vi "Goal-directed Line Following.vi"() -> ()   [LabVIEW 2019]
uses:
  SubVIs/GDLF SM States.ctl
  <vilib>/Platform/TimedLoop/XDataNode/timing_clust.ctl
  <vilib>/Platform/TimedLoop/XDataNode/nitl_modes.ctl
  <vilib>/Platform/TimedLoop/XDataNode/wakeup.ctl
  <extravilib>/ChannelInstances/Tag-bool/Write With Abort.vi
  <extravilib>/ChannelInstances/Tag-a[.](dbl)/Read With Abort.vi
  <extravilib>/ChannelInstances/Tag-a[.](dbl)/Write With Abort.vi
  <extravilib>/ChannelInstances/Tag-bool/Read With Abort.vi
  <extravilib>/ChannelInstances/Tag-dbl/Write With Abort.vi
  <extravilib>/ChannelInstances/Lossy Stream-a[.,.](dbl)/Read With Abort.vi
  <extravilib>/ChannelInstances/Tag-dbl/Read With Abort.vi
  <extravilib>/ChannelInstances/Lossy Stream-a[.,.](dbl)/Write With Abort.vi
  <extravilib>/ChannelInstances/Lossy Stream-a[.,.](dbl)/EndpointRead.vi
  <extravilib>/ChannelInstances/Lossy Stream-a[.,.](dbl)/Endpoint.vi
  <extravilib>/ChannelInstances/Tag-bool/Instantiate.vi
  <extravilib>/ChannelInstances/Tag-dbl/Instantiate.vi
  <extravilib>/ChannelInstances/Lossy Stream-a[.,.](dbl)/Instantiate.vi
  <extravilib>/ChannelInstances/Tag-a[.](dbl)/Instantiate.vi
  <extravilib>/ChannelInstances/Tag-bool/EndpointRead.vi
  <extravilib>/ChannelInstances/Tag-a[.](dbl)/EndpointRead.vi
  <extravilib>/ChannelInstances/Tag-dbl/EndpointRead.vi
  <extravilib>/ChannelInstances/Lossy Stream-a[.,.](dbl)/)Channel.vi
  <extravilib>/ChannelInstances/Tag-bool/Endpoint.vi
  <extravilib>/ChannelInstances/Tag-a[.](dbl)/Endpoint.vi
  <extravilib>/ChannelInstances/Tag-dbl/Endpoint.vi
  <resource>/ChannelSupport/_ChannelSupport/WaitIfNeeded.vi
  <vilib>/Platform/TimedLoop/XDataNode/XDataNode.xnode
  <extravilib>/ChannelInstances/Tag-bool.lvlib
  <vilib>/Platform/TimedLoop/XDataNode/XDNodeRunTimeDep.lvlib
  <extravilib>/ChannelInstances/Tag-a[.](dbl).lvlib
  <extravilib>/ChannelInstances/Lossy Stream-a[.,.](dbl).lvlib
  <extravilib>/ChannelInstances/Tag-dbl.lvlib
panel:
  in  "Hue Threshold":cluster{i32, i32}(slide)={0, 255} scale=0.0..255.0
  in  "Saturation Threshold":cluster{i32, i32}(slide)={0, 255} scale=0.0..255.0
  in  "Luminance Threshold":cluster{i32, i32}(slide)={0, 255} scale=0.0..255.0
  out "error out":errorcluster
  out "System State":T1
  out "Destination Task \nCoordinates (cm)":dbl[](array[numeric])
  in  "Stop Button":bool
  out "Calibrated":bool
  out "Information":string
  in  "GO?":bool
  out "Processed Image":T2(plugin-control)
  out "Desired Task \nCoordinates (cm)":dbl[](array[numeric])
  out "Current Task Coordinates (cm)":dbl[](array[numeric])
  out "Silk":T2(plugin-control)
  out "Original Acquired Image":T2(plugin-control)
  # "Mechatronic Systems Board"
  # "Goal-directed Line Following"
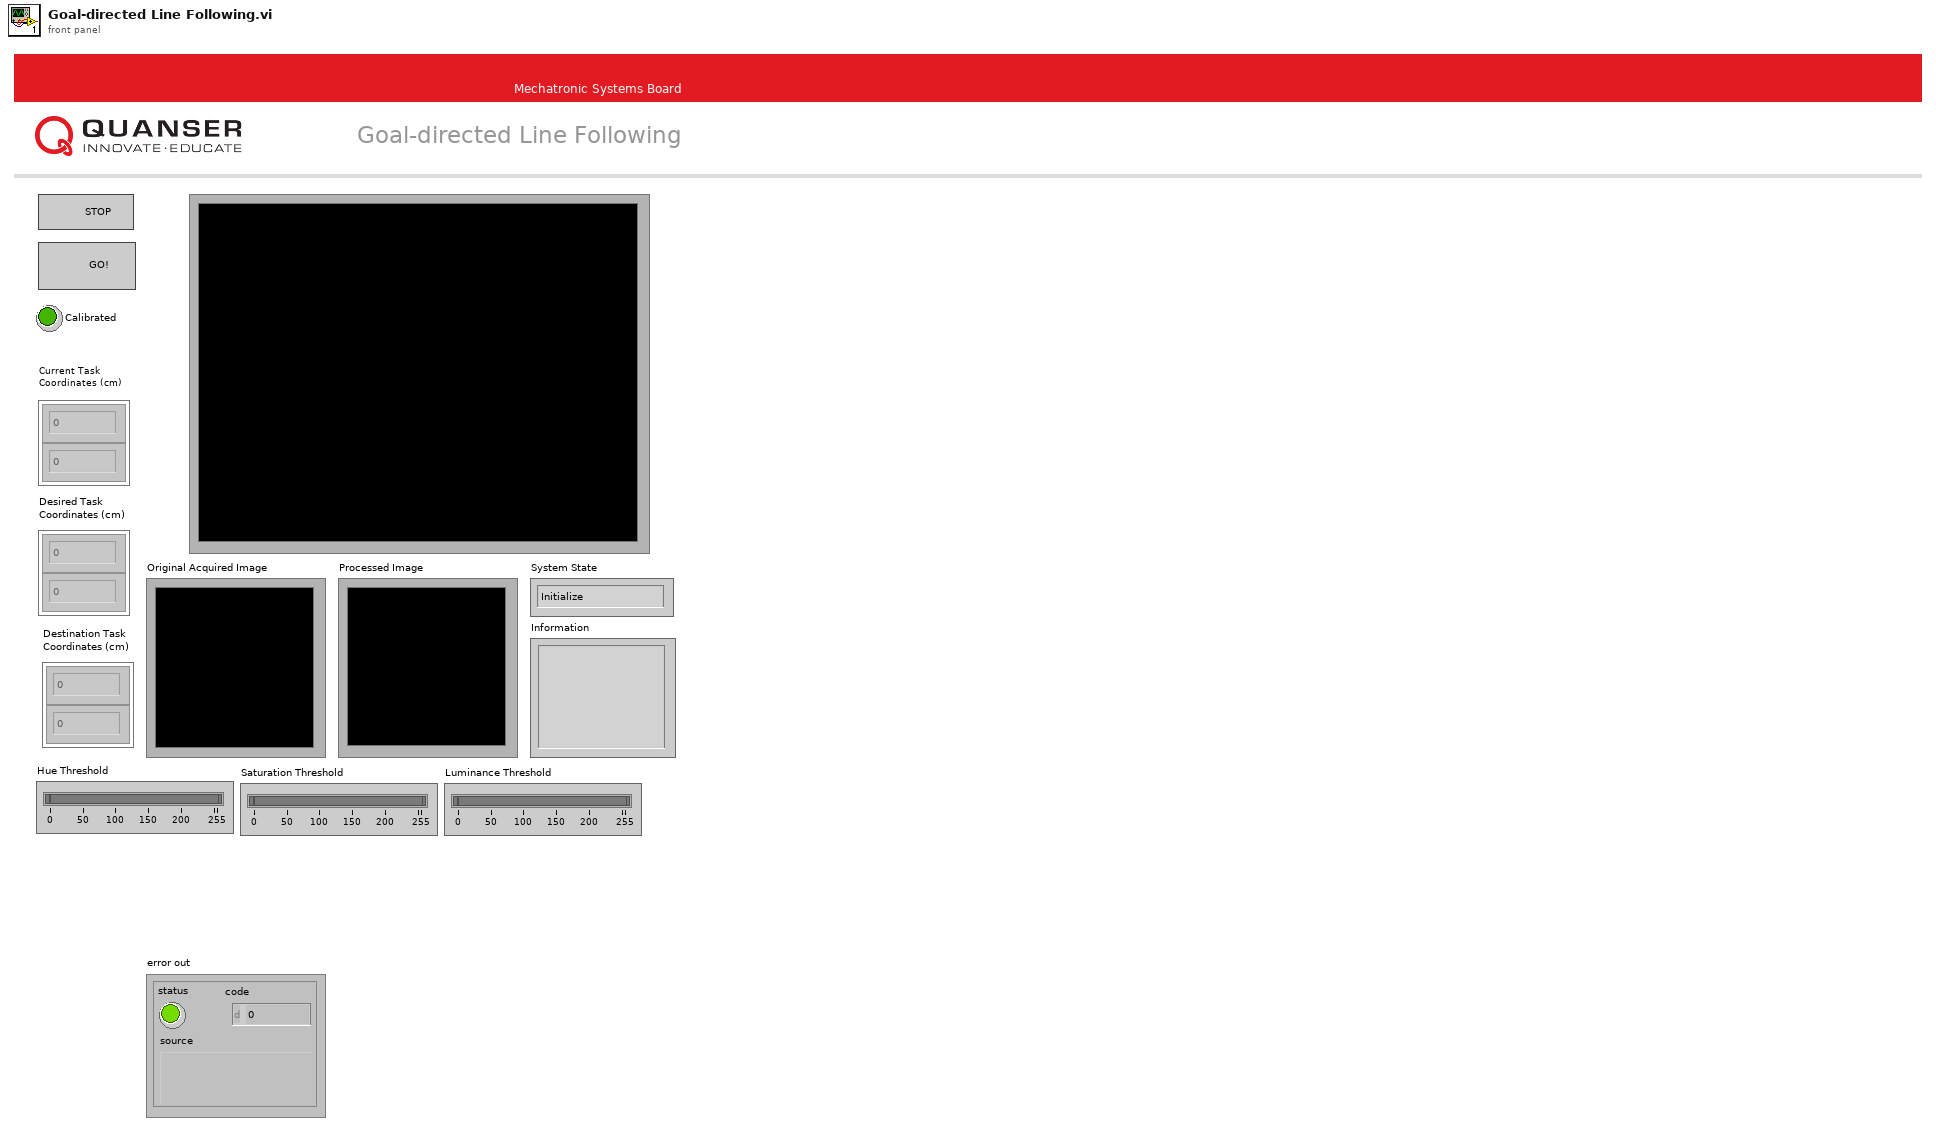
[diagram p1: front panel]
types:
  T1 = typedef "GDLF SM States.ctl" = enum16{"Initialize", "Set Destination", "Move", "Wait", "Backtrack", "Stop"}
  T2 = typedef "IMAQ Image.ctl" = refnum<image>
  T3 = typedef "QNET MS IO Cluster.ctl" = cluster{"Error":errorcluster, "Encoder Calibration Values":i32[], "Update Calibration":bool, "JPEG Resolutions":u16, "Raw Resolutions":u16, "Image Mode":enum16{"RAW RGB", "RAW Gray Scale", "JPEG"}, "FPGA Ref":refnum<k20>}
  T4 = typedef "XDNodeRunTimeDep.lvlib/timing_clust.ctl" = cluster{"Expected End [f-1]":u64, "Actual End [f-1]":u64, "Finished Late? [f-1]":bool, "Expected End [i-1]":u64, "Actual End [i-1]":u64, "Finished Late? [i-1]":bool, "Expected Start [i]":u64, "Actual Start [i]":u64, "Expected Start [f]":u64, "Actual Start [f]":u64, "Source Name":string, "Structure Name":string, "Period":i64, "Deadline":i64, "Offset":i64, "Start":i64, "Priority":i32, "Timeout":i32, "Mode":T5, "Wakeup Reason":T6, "Error":errorcluster, "Source Type":string, "Secondary Source Type":string, "Global End Time":u64, "Global Start Time":u64, "Frame Duration":u64, "Iteration Duration":u64, "Assigned CPU":i32, "I/O Scan Engine Mode":u32}
  T5 = typedef "XDNodeRunTimeDep.lvlib/nitl_modes.ctl" = enum32{"No Change", "Process missed periods, maintain original phase", "Discard missed periods, maintain original phase", "Process missed periods, ignore original phase", "Discard missed periods, ignore original phase"}
  T6 = typedef "XDNodeRunTimeDep.lvlib/wakeup.ctl" = enum32{"Normal", "Aborted", "Asynchronous wakeup", "Timing source error", "Timed loop error", "Timeout"}
  T7 = typedef "ROI Descriptor" = cluster{"Global Rectangle":i32[], "Contours":cluster{"ID":enum32{"External", "Internal"}, "Type":u32, "Coordinates":i32[]}[]}
  T8 = cluster{"Hue Threshold":cluster{i32, i32}, "Saturation Threshold":cluster{i32, i32}, "Luminance Threshold":cluster{i32, i32}}
  T9 = typedef "Lossy Stream-a[.,.](dbl).lvlib/)Channel.ctl" = refnum<queue>
  T10 = typedef "Tag-a[.](dbl).lvlib/))Channel.ctl" = refnum<queue>
  T11 = typedef "Tag-bool.lvlib/))Channel.ctl" = refnum<queue>
  T12 = cluster{"Global Rectangle":i32[], "Contours":cluster{"Contour Type":u32, "ROI Type":u32, "Points":i32[]}[]}
  T13 = typedef "Tag-dbl.lvlib/))Channel.ctl" = refnum<queue>
  T14 = cluster{"Contour Type":u32, "ROI Type":u32, "Points":i32[]}[]
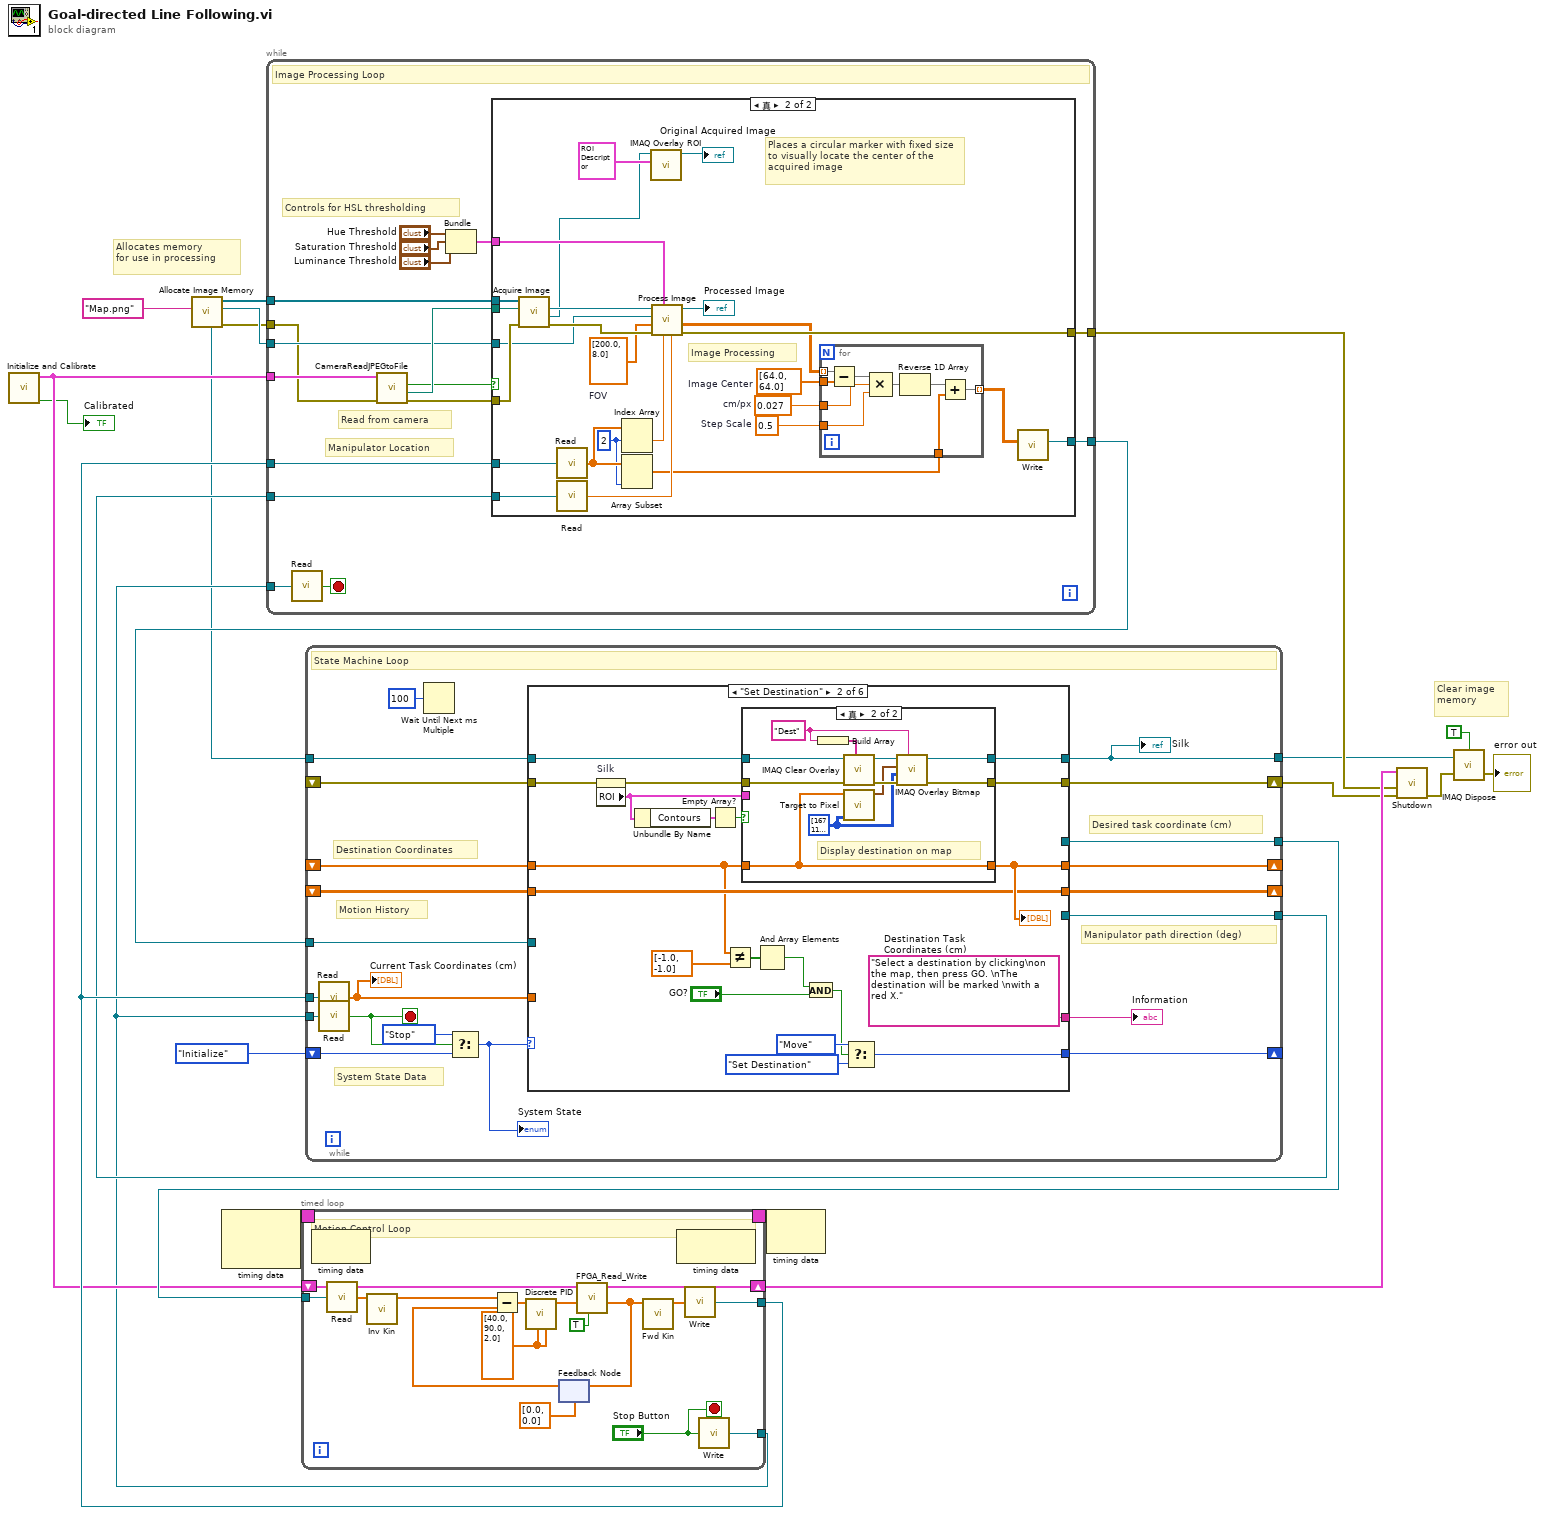
[diagram p0: block diagram]
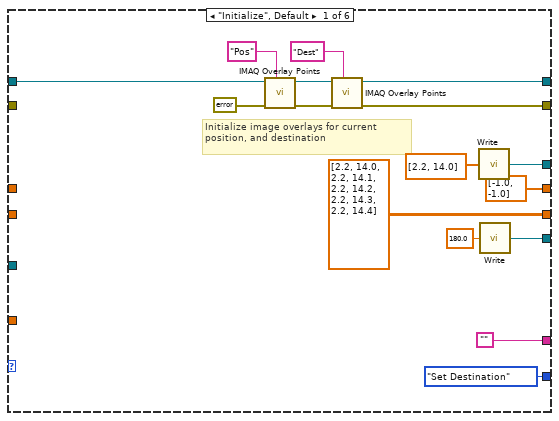
[diagram p2: hidden frame]
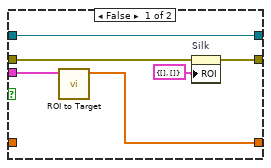
[diagram p3: hidden frame]
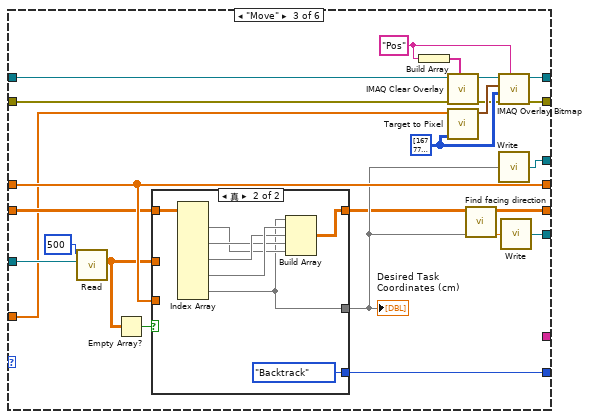
[diagram p4: hidden frame]
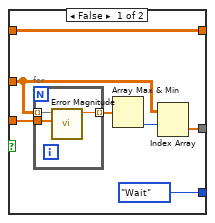
[diagram p5: hidden frame]
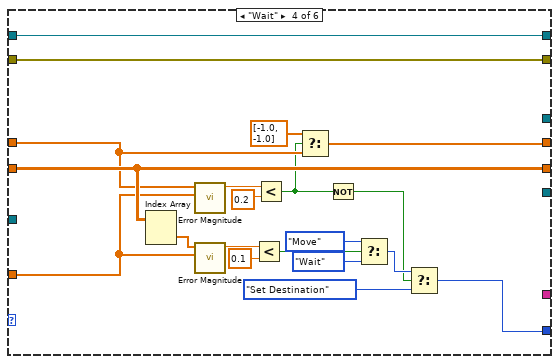
[diagram p6: hidden frame]
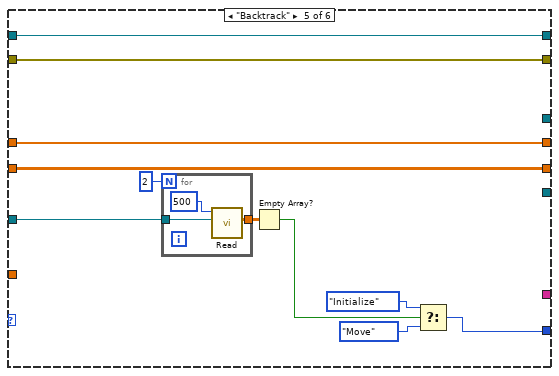
[diagram p7: hidden frame]
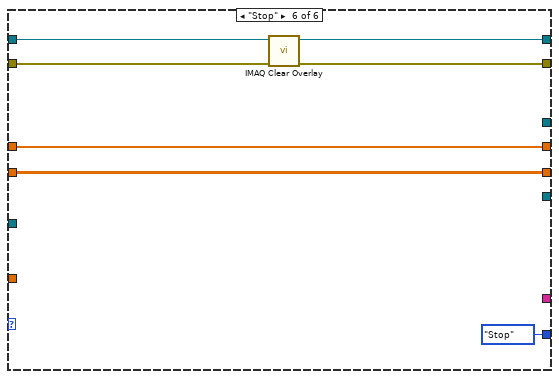
[diagram p8: hidden frame]
diagram:
  # "Allocates memory\nfor use in processing"
  # "Clear image\nmemory"
  n1 = call "Initialize and Calibrate.vi"() -> ("Calibrated"=→"Calibrated":bool, "IO Cluster"=w11:T3)  [unwired: 10 in]
  n2 = call "Allocate Image Memory.vi"("Base Image File"="Map.png") -> ("error out"=w19:errorcluster, "HSL Threshold"=w20:T2, "Acquisition Memory"=w21:T2[], "Base Image"=w2:T2)  [unwired: 5 in, 2 out]
  n3 = node-c288() -> (w18:T4)  [unwired: 2 in]
  n4 = while {
    tunnel: w11 -> [w39]
    tunnel: [w35] -> w8
    tunnel: w21 -> [w34]
    tunnel: w20 -> [w33]
    tunnel: w19 -> [w32]
    tunnel: [w31] -> w14
    tunnel: w15 -> [w29]
    tunnel: w13 -> [w30]
    tunnel: w4 -> [w28]
    stop <- w27 stop-if-true
    # "Controls for HSL thresholding"
    # "Read from camera"
    # "Manipulator Location"
    # "Image Processing Loop"
    n5 = call <extravilib>:"Read.vi"("channel"=w28) -> ("element"=w27:bool)  [unwired: 1 in, 1 out]
    n6 = call "CameraReadJPEGtoFile.vi"("error in"=w32, "IO Cluster In"=w39) -> ("Error Out"=w36:errorcluster, "Image File"=w38:path, "New Image Data"=w37:bool)  [unwired: 6 in, 1 out]
    n7 = Bundle("Hue Threshold"="Hue Threshold", "Saturation Threshold"="Saturation Threshold", "Luminance Threshold"="Luminance Threshold") -> (w23:T8)  [unwired: 1 in]
    n8 = case shown="真" w37 {
      tunnel: w38 -> [_ w64]
      tunnel: w36 -> [w40 w65]
      tunnel: [w40 w60] -> w35
      tunnel: w34 -> [_ w63]
      tunnel: w33 -> [_ w55]
      tunnel: [_ w52] -> w31
      tunnel: w30 -> [_ w46]
      tunnel: w29 -> [_ w45]
      tunnel: w23 -> [_ w44]
      frame False {
      }
      frame True {
        w50 = 2 ("index")
        w53 = 0.5  # Step Scale
        w58 = 0.027  # cm/px
        w57 = dbl[] [64.0, 64.0]  # Image Center
        w59 = dbl[] [200.0, 8.0]  # FOV
        # "Image Processing"
        # "Places a circular marker with fixed size to visually locate the center of the acquired image"
        n9 = call "Acquire Image.vi"("Error In"=w65, "File Path"=w64, "Acquisition Memory"=w63) -> ("Error Out"=w61:errorcluster, "Source Image"=w41:T2, "HSL Image"=w42:T2)  [unwired: 4 in, 2 out]
        n10 = call <extravilib>:"Read.vi"("channel"=w45) -> ("element"=w51:dbl[])  [unwired: 1 in, 1 out]
        n11 = call <extravilib>:"Read.vi"("channel"=w46) -> ("element"=w49:dbl)  [unwired: 1 in, 1 out]
        n12 = Index Array(array=w51, index #1=w50) -> (element #1=w48:dbl)  [unwired: 1 in, 1 out]
        n13 = Array Subset(array=w51, length=w50) -> (w47:dbl[])  [unwired: 1 in]
        n14 = call "IMAQ Overlay ROI"("ROI Descriptor"=T7 {"Global Rectangle"=[16, 0, 145, 129], "Contours"=[{"ID"=enum."External", "Type"=7, "Coordinates"=[64, 64, 7, 8, 0, 0]}]}, "Image"=w41) -> ("Image Out"=→"Original Acquired Image":T2)  [unwired: 8 in, 1 out]
        n15 = call "Process Image.vi"("Path Angle"=w49, "Camera Angle"=w48, 7:w44, "Error In"=w61, "FOV"=w59, "Process Memory"=w55, "Acquired Image"=w42) -> ("Error Out"=w60:errorcluster, "Particle Locations"=w56:dbl[][], "Processed Image"=→"Processed Image":T2)  [unwired: 2 in]
        n16 = for {
          tunnel: w57 -> [w75]
          tunnel: [w73] -> w54 mode=indexing
          tunnel: w56 -> [w72] mode=indexing
          tunnel: w58 -> [w71]
          tunnel: w47 -> [w68]
          tunnel: w53 -> [w67]
          n17 = Subtract(x=w72, y=w75) -> (x-y=w74:dbl[])
          n18 = Compound Arithmetic op=MULTIPLY(w74, w71, w67) -> (w70:dbl[])
          n19 = Reverse 1D Array(array=w70) -> (reversed array=w69:dbl[])
          n20 = Add(x=w69, y=w68) -> (x+y=w73:dbl[])
        }
        n21 = call <extravilib>:"Write.vi"("element"=w54) -> ("channel"=w52:T9)  [unwired: 8 in, 2 out]
      }
    }
  }
  n22 = timed-loop {
    timing: w18 -> [_]
    timing-out: [_] -> w17
    tunnel: [w82] -> w15
    tunnel: w16 -> [w81]
    shift-right: [w87] -> w12
    shift-left: w11 -> [w79]
    tunnel: [w77] -> w4
    stop <- "Stop Button" stop-if-true
    w76 = dbl[] [40.0, 90.0, 2.0] ("Gains Motor 0")
    # "Motion Control Loop"
    n23 = node-c288() -> ()  [unwired: 1 in, 1 out]
    n24 = call <extravilib>:"Read.vi"("channel"=w81) -> ("element"=w80:dbl[])  [unwired: 1 in, 1 out]
    n25 = call "Inv Kin.vi"("Task Coordinates (cm)"=w80) -> ("Joint Coordinates (rad)"=w88:dbl[])  [unwired: 10 in]
    n26 = feedback #1(dbl[] [0.0, 0.0] ("Joint Coordinates (rad)")) -> (w86:dbl[])
    n27 = Subtract(x=w88, y=w86) -> (x-y=w89:dbl[])
    n28 = call "Discrete PID.vi"("Gains Motor 1"=w76, "Gains Motor 0"=w76, "Error Array"=w89) -> ("Voltage"=w90:dbl[])  [unwired: 8 in]
    n29 = call "FPGA_Read_Write.vi"("Motors enabled?"=TRUE, "Commands"=w90, "IO Cluster In"=w79) -> ("Joint Coordinates (rad)"=w85:dbl[], "IO Cluster Out"=w87:T3)  [unwired: 5 in, 2 out]
    n30 = feedback-in #1(w85) -> ()
    n31 = call "Fwd Kin.vi"("Joint Coordinates (rad)"=w85) -> ("Task Coordinates (cm)"=w83:dbl[])  [unwired: 9 in, 1 out]
    n32 = node-c288() -> ()  [unwired: 1 in, 1 out]
    n33 = call <extravilib>:"Write.vi"("element"=w83) -> ("channel"=w82:T10)  [unwired: 1 out]
    n34 = call <extravilib>:"Write.vi"("element"="Stop Button") -> ("channel"=w77:T11)  [unwired: 1 out]
  }
  n35 = while {
    tunnel: w4 -> [w114]
    shift-right: [w112] -> _
    shift-left: _ -> [w113]
    tunnel: w14 -> [w109]
    tunnel: [w105] -> w16
    tunnel: w15 -> [w111]
    tunnel: [w106] -> w13
    tunnel: w2 -> [w104]
    shift-right: [w108] -> _
    shift-left: _ -> [w107]
    shift-right: [w103] -> _
    shift-left: GDLF_SM_States."Initialize" ("System State") -> [w101]
    shift-right: [w97] -> w9
    shift-left: _ -> [w96]
    tunnel: [w94] -> w6
    stop <- w98 stop-if-true
    # "Manipulator path direction (deg)"
    # "Destination Coordinates"
    # "Motion History"
    # "Desired task coordinate (cm)"
    # "System State Data"
    # "State Machine Loop"
    n36 = call <extravilib>:"Read.vi"("channel"=w111) -> ("element"=w110:dbl[])  [unwired: 1 in, 1 out]
    "Current Task Coordinates (cm)" <- w110
    n37 = call <extravilib>:"Read.vi"("channel"=w114) -> ("element"=w98:bool)  [unwired: 1 in, 1 out]
    n38 = Wait Until Next ms Multiple(millisecond multiple=u32 100) -> ()  [unwired: 1 out]
    n39 = Select(t=GDLF_SM_States."Stop", s=w98, f=w101) -> (s? t:f=w100:T1)
    "System State" <- w100
    n40 = case shown="\"Set Destination\"" w100 {
      tunnel: w113 -> [_ w145 w173 w226 w237 w249]
      tunnel: [dbl[][] [[2.2, 14.0], [2.2, 14.1], [2.2, 14.2], [2.2, 14.3], [2.2, 14.4]] w145 w177 w226 w237 w249] -> w112
      tunnel: w110 -> [_ _ w168 w215 _ _]
      tunnel: w107 -> [_ w137 w184 w218 w239 w248]
      tunnel: w109 -> [_ _ w191 _ w235 _]
      tunnel: [dbl[] [-1.0, -1.0] ("Joint Coordinates (rad)") w150 w184 w217 w239 w248] -> w108
      tunnel: [w127 _ w190 _ _ _] -> w106
      tunnel: [w124 _ w189 _ _ _] -> w105
      tunnel: w104 -> [w122 w144 w188 w219 w238 w247]
      tunnel: [GDLF_SM_States."Set Destination" ("System State") w149 w171 w210 w230 GDLF_SM_States."Stop" ("System State")] -> w103
      tunnel: ["" "Select a destination by clicking\non the map, then press GO. \nThe destination will be marked \nwith a red X." _ _ _ _] -> w102
      tunnel: [w117 w142 w185 w220 w240 w244] -> w97
      tunnel: w96 -> [_ w146 w187 w220 w240 w246]
      tunnel: [w119 w141 w186 w219 w238 w245] -> w94
      frame "Initialize", Default {
        # "Initialize image overlays for current\nposition, and destination"
        n41 = call "IMAQ Overlay Points"("Group"="Pos", "error in (no error)"=errorcluster {"status"=FALSE, "code"=0, "source"=""} ("error out"), "Image"=w122) -> ("error out"=w118:errorcluster, "Image Out"=w120:T2)  [unwired: 7 in]
        n42 = call "IMAQ Overlay Points"("Group"="Dest", "error in (no error)"=w118, "Image"=w120) -> ("error out"=w117:errorcluster, "Image Out"=w119:T2)  [unwired: 7 in]
        n43 = call <extravilib>:"Write.vi"("element"=dbl[] [2.2, 14.0] ("Joint Coordinates (rad)")) -> ("channel"=w124:T10)  [unwired: 1 out]
        n44 = call <extravilib>:"Write.vi"("element"=180.0) -> ("channel"=w127:T13)  [unwired: 1 out]
      }
      frame "Set Destination" {
        n45 = property on="Silk" class="ImageControl"(error in=w146) -> (error out=w143:errorcluster, "ROI"=w138:T12)  [unwired: 1 in, 1 out]
        n46 = Unbundle By Name(w138) -> ("Contours"=w139:T14)
        n47 = Empty Array?(array=w139) -> (empty?=w140:bool)
        n48 = Not Equal?(x=w137, y=dbl[] [-1.0, -1.0] ("Joint Coordinates (rad)")) -> (x != y?=w133:bool[])
        n49 = case shown="真" w140 {
          tunnel: [w151 w163] -> w150
          tunnel: w144 -> [w153 w165]
          tunnel: w143 -> [w152 w160]
          tunnel: [w155 w159] -> w142
          tunnel: [w153 w164] -> w141
          tunnel: w137 -> [_ w163]
          tunnel: w138 -> [w156 _]
          frame False {
            n50 = call "ROI to Target.vi"("ROI"=w156) -> ("Target Coordinates"=w151:dbl[])  [unwired: 8 in, 2 out]
            n51 = property on="Silk" class="ImageControl"(error in=w152, "ROI"=T12 {"Global Rectangle"=[], "Contours"=[]}) -> (error out=w155:errorcluster)  [unwired: 1 in, 1 out]
          }
          frame True {
            w158 = "Dest" ("Group")
            w161 = u32[][] [[16711680, 16711680, 16777216, 16777216, 16777216, 16777216, 16777216, 16711680, 16711680], [16711680, 16711680, 16711680, 16777216, 16777216, 16777216, 16711680, 16711680, 16711680], [16777216, 16711680, 16711680, 16711680, 16777216, 16711680, 16711680, 16711680, 16777216], [16777216, 16777216, 16711680, 16711680, 16711680, 16711680, 16711680, 16777216, 16777216], [16777216, 16777216, 16777216, 16711680, 16711680, 16711680, 16777216, 16777216, 16777216], [16777216, 16777216, 16711680, 16711680, 16711680, 16711680, 16711680, 16777216, 16777216], [16777216, 16711680, 16711680, 16711680, 16777216, 16711680, 16711680, 16711680, 16777216], [16711680, 16711680, 16711680, 16777216, 16777216, 16777216, 16711680, 16711680, 16711680], [16711680, 16711680, 16777216, 16777216, 16777216, 16777216, 16777216, 16711680, 16711680]] ("Bitmap")
            # "Display destination on map"
            n52 = Build Array(w158) -> (w157:string[])
            n53 = call "IMAQ Clear Overlay"("Groups"=w157, "error in (no error)"=w160, "Image"=w165) -> ("error out"=w166:errorcluster, "Image Out"=w167:T2)  [unwired: 7 in]
            n54 = call "Target to Pixel.vi"("Symbol"=w161, "Target Coordinates"=w163) -> ("Target Pixel"=w162:cluster{"X":i32, "Y":i32})  [unwired: 9 in]
            n55 = call "IMAQ Overlay Bitmap"("Group"=w158, "error in (no error)"=w166, "Bitmap"=w161, "Top Left Point"=w162, "Image"=w167) -> ("error out"=w159:errorcluster, "Image Out"=w164:T2)  [unwired: 5 in]
          }
        }
        "Destination Task \nCoordinates (cm)" <- w150
        n56 = And Array Elements(Boolean array=w133) -> (logical AND=w132:bool)
        n57 = And(x=w132, y="GO?") -> (x .and. y?=w134:bool)
        n58 = Select(t=GDLF_SM_States."Move" ("System State"), s=w134, f=GDLF_SM_States."Set Destination" ("System State")) -> (s? t:f=w149:T1)
      }
      frame "Move" {
        w179 = "Pos" ("Group")
        w182 = u32[][] [[16777216, 16777216, 6618880, 16777216, 6618880, 16777216, 6618880, 16777216, 16777216], [16777216, 6618880, 16777216, 6618880, 16777216, 6618880, 16777216, 6618880, 16777216], [6618880, 16777216, 6618880, 16777216, 6618880, 16777216, 6618880, 16777216, 6618880], [16777216, 6618880, 16777216, 6618880, 16777216, 6618880, 16777216, 6618880, 16777216], [6618880, 16777216, 6618880, 16777216, 6618880, 16777216, 6618880, 16777216, 6618880], [16777216, 6618880, 16777216, 6618880, 16777216, 6618880, 16777216, 6618880, 16777216], [6618880, 16777216, 6618880, 16777216, 6618880, 16777216, 6618880, 16777216, 6618880], [16777216, 6618880, 16777216, 6618880, 16777216, 6618880, 16777216, 6618880, 16777216], [16777216, 16777216, 6618880, 16777216, 6618880, 16777216, 6618880, 16777216, 16777216]] ("Bitmap")
        n59 = call <extravilib>:"Read.vi"("channel"=w191, "timeout in ms (-1)"=500) -> ("element"=w174:dbl[][])  [unwired: 4 in, 5 out]
        n60 = Empty Array?(array=w174) -> (empty?=w169:bool)
        n61 = case shown="真" w169 {
          tunnel: w174 -> [w196 _]
          tunnel: w184 -> [w195 _]
          tunnel: [w194 w203] -> w175
          tunnel: w173 -> [w193 w208]
          tunnel: [w193 w202] -> w172
          tunnel: [GDLF_SM_States."Wait" ("System State") GDLF_SM_States."Backtrack" ("System State")] -> w171
          frame False {
            n62 = for {
              tunnel: w196 -> [w201] mode=indexing
              tunnel: [w200] -> w198 mode=indexing
              tunnel: w195 -> [w199]
              n63 = call "Error Magnitude.vi"("Actual Task Coordinates (cm)"=w199, "Desired Task Coordinates (cm)"=w201) -> ("Task-space\nError"=w200:dbl)  [unwired: 9 in]
            }
            n64 = Array Max & Min(array=w198) -> (min index (indices)=w197:i32)  [unwired: 3 out]
            n65 = Index Array(array=w196, index (row)=w197) -> (element=w194:dbl[])  [unwired: 1 in]
          }
          frame True {
            n66 = Index Array(array=w208) -> (element #1=w204:dbl[], element #2=w205:dbl[], element #3=w206:dbl[], element #4=w207:dbl[], element #5=w203:dbl[])  [unwired: 10 in]
            n67 = Build Array(w203, w207, w206, w205, w204) -> (w202:dbl[][])
          }
        }
        "Desired Task \nCoordinates (cm)" <- w175
        n68 = Build Array(w179) -> (w178:string[])
        n69 = call "IMAQ Clear Overlay"("Groups"=w178, "error in (no error)"=w187, "Image"=w188) -> ("error out"=w180:errorcluster, "Image Out"=w181:T2)  [unwired: 7 in]
        n70 = call "Target to Pixel.vi"("Symbol"=w182, "Target Coordinates"=w168) -> ("Target Pixel"=w183:cluster{"X":i32, "Y":i32})  [unwired: 9 in]
        n71 = call "Find facing direction.vi"("Desired Task Coordinates (cm)"=w175, "Motion History In"=w172) -> ("Facing Direction (deg)"=w176:dbl, "Motion History Out"=w177:dbl[][])  [unwired: 8 in]
        n72 = call "IMAQ Overlay Bitmap"("Group"=w179, "error in (no error)"=w180, "Bitmap"=w182, "Top Left Point"=w183, "Image"=w181) -> ("error out"=w185:errorcluster, "Image Out"=w186:T2)  [unwired: 5 in]
        n73 = call <extravilib>:"Write.vi"("element"=w175) -> ("channel"=w189:T10)  [unwired: 1 out]
        n74 = call <extravilib>:"Write.vi"("element"=w176) -> ("channel"=w190:T13)  [unwired: 1 out]
      }
      frame "Wait" {
        n75 = Index Array(array=w226) -> (element=w229:dbl[])  [unwired: 2 in]
        n76 = call "Error Magnitude.vi"("Actual Task Coordinates (cm)"=w215, "Desired Task Coordinates (cm)"=w218) -> ("Task-space\nError"=w222:dbl)  [unwired: 9 in]
        n77 = call "Error Magnitude.vi"("Actual Task Coordinates (cm)"=w215, "Desired Task Coordinates (cm)"=w229) -> ("Task-space\nError"=w228:dbl)  [unwired: 9 in]
        n78 = Less?(x=w228, y=0.1) -> (x < y?=w224:bool)
        n79 = Less?(x=w222, y=0.2) -> (x < y?=w212:bool)
        n80 = Select(t=dbl[] [-1.0, -1.0], s=w212, f=w218) -> (s? t:f=w217:dbl[])
        n81 = Not(x=w212) -> (.not. x?=w211:bool)
        n82 = Select(t=GDLF_SM_States."Move", s=w224, f=GDLF_SM_States."Wait") -> (s? t:f=w214:T1)
        n83 = Select(t=w214, s=w211, f=GDLF_SM_States."Set Destination" ("t")) -> (s? t:f=w210:T1)
      }
      frame "Backtrack" {
        n84 = for {
          N: 2 -> [_]
          tunnel: w235 -> [w243]
          tunnel: [w242] -> w234
          n85 = call <extravilib>:"Read.vi"("channel"=w243, "timeout in ms (-1)"=500) -> ("element"=w242:dbl[][])  [unwired: 4 in, 5 out]
        }
        n86 = Empty Array?(array=w234) -> (empty?=w233:bool)
        n87 = Select(t=GDLF_SM_States."Initialize" ("System State"), s=w233, f=GDLF_SM_States."Move") -> (s? t:f=w230:T1)
      }
      frame "Stop" {
        n88 = call "IMAQ Clear Overlay"("error in (no error)"=w246, "Image"=w247) -> ("error out"=w244:errorcluster, "Image Out"=w245:T2)  [unwired: 8 in]
      }
    }
    "Information" <- w102
    "Silk" <- w94
  }
  n89 = node-c288(w17) -> ()  [unwired: 1 out]
  n90 = call "Shutdown.vi"("Image Processing Loop"=w9, "Manipulator Loop"=w8, "IO Cluster In"=w12) -> ("Error"=w7:errorcluster)  [unwired: 8 in]
  n91 = call "IMAQ Dispose"("All Images? (No)"=TRUE, "Image"=w6, "error in (no error)"=w7) -> ("error out"=→"error out":errorcluster)  [unwired: 3 in]
